vi "test_count.vi"() -> ()   [LabVIEW 2013]
uses:
  <vilib>/rvi/FXPMathLib/FxpSub/XNode/nifxpmath_Sub.xnode
  <vilib>/rvi/FXPMathLib/sim/FxpSim.dll
panel:
  out "Waveform Graph 3":i16[](graph)
  out "Waveform Graph 2":i16[](graph)
  out "counting":bool
  out "output valid":bool
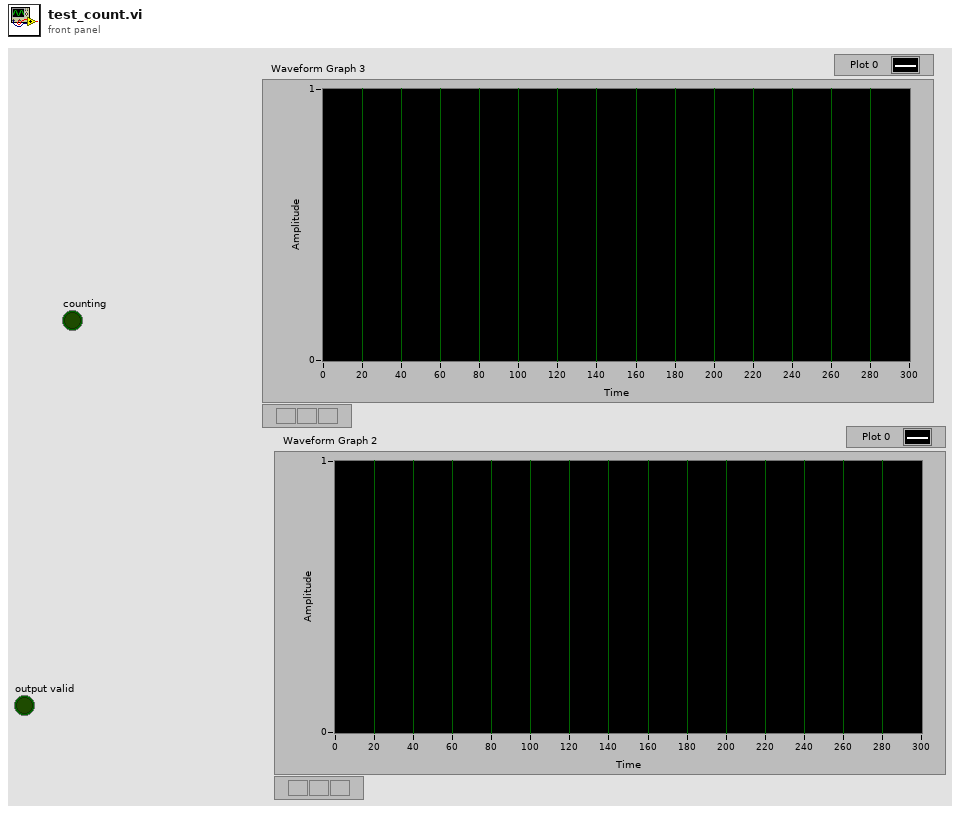
[diagram p1: front panel]
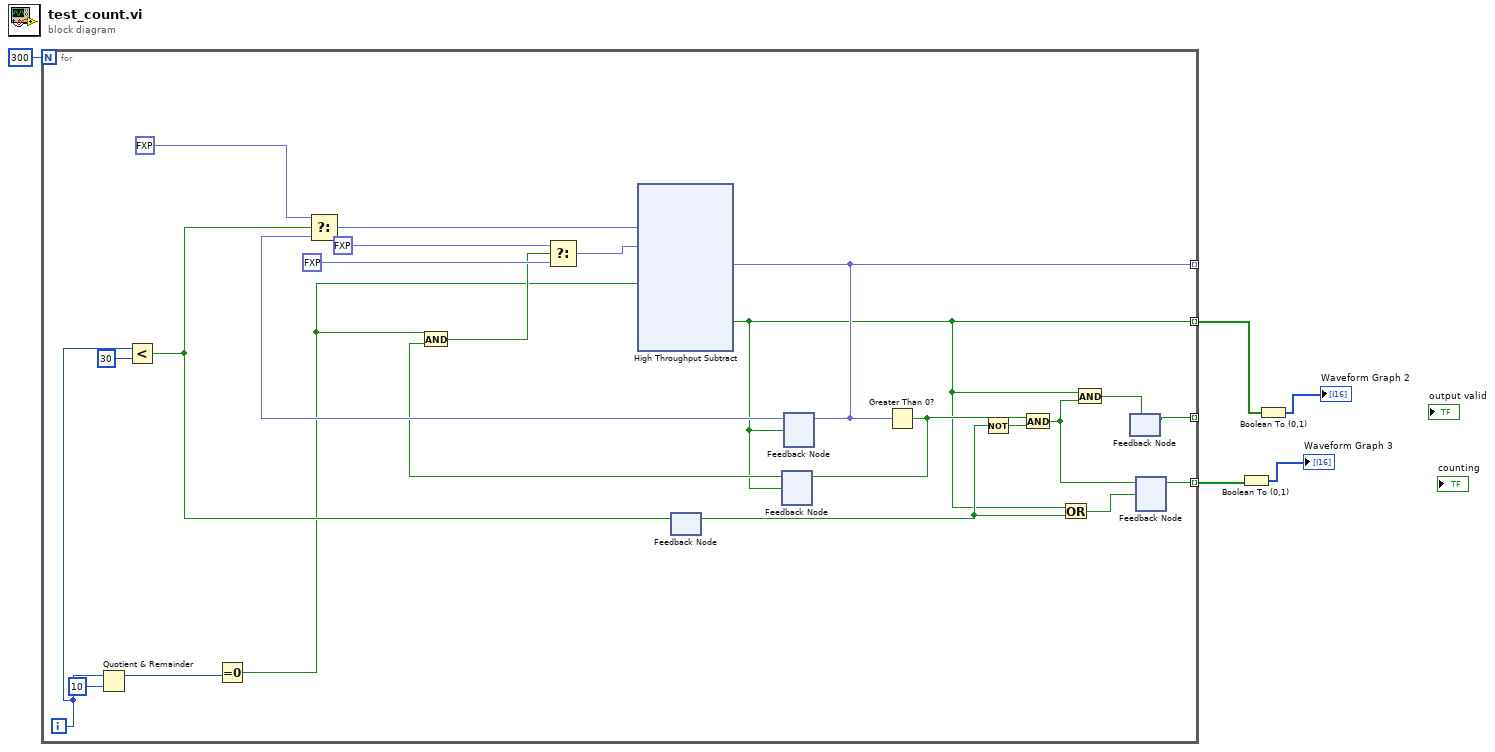
[diagram p0: block diagram]
diagram:
  n1 = for {
    N: 300 -> [_]
    tunnel: [w9] -> _ mode=indexing
    tunnel: [w8] -> w3 mode=indexing
    tunnel: [w7] -> _ mode=indexing
    tunnel: [w6] -> w2 mode=indexing
    i -> [w14]
    n2 = Quotient & Remainder(x=w14, y=10) -> (x-y*floor(x/y)=w11:i32)  [unwired: 1 out]
    n3 = Less?(x=w14, y=30) -> (x < y?=w12:bool)
    n4 = Equal To 0?(x=w11) -> (x = 0?=w10:bool)
    n5 = feedback #1() -> (w19:bool)  [unwired: 1 in]
    n6 = feedback-in #1(w12) -> ()
    n7 = feedback #2() -> (w21:bool)  [unwired: 1 in]
    n8 = And(x=w10, y=w21) -> (x .and. y?=w20:bool)
    n9 = Select(t=fxp<+,16,16> 1.0 ("y"), s=w20, f=fxp<+,16,16> 0.0 ("y")) -> (s? t:f=w24:fxp<+,16,16>)
    n10 = feedback #3() -> (w25:fxp<+,16,16>)  [unwired: 1 in]
    n11 = Select(t=fxp<+,16,16> 15.0 ("Samples to count"), s=w12, f=w25) -> (s? t:f=w28:fxp<+,16,16>)
    n12 = xnode "High Throughput Subtract"("x"=w28, "y"=w24, "input valid"=w10) -> ("x-y"=w7:fxp<+,16,16>, "output valid"=w6:bool)  [unwired: 1 in, 1 out]
    n13 = feedback-in #3(w7, w6) -> ()
    n14 = Greater Than 0?(x=w7) -> (x > 0?=w17:bool)
    n15 = feedback-in #2(w17, w6) -> ()
    n16 = Not(x=w19) -> (.not. x?=w18:bool)
    n17 = And(x=w17, y=w18) -> (x .and. y?=w16:bool)
    n18 = Or(x=w6, y=w19) -> (x .or. y?=w22:bool)
    n19 = And(x=w6, y=w16) -> (x .and. y?=w23:bool)
    n20 = feedback #4() -> (w9:bool)  [unwired: 1 in]
    n21 = feedback-in #4(w23) -> ()
    n22 = feedback #5() -> (w8:bool)  [unwired: 1 in]
    n23 = feedback-in #5(w16, w22) -> ()
  }
  n24 = Boolean To (0,1)(Boolean=w3) -> (0, 1=→"Waveform Graph 3":i16[])
  n25 = Boolean To (0,1)(Boolean=w2) -> (0, 1=→"Waveform Graph 2":i16[])
